vi "EQC LoadFile PixelReg.vi"(11 "PixelReg file path":path) -> (0 "Error tick":bool, 2 "PixelReg (hex)":u32[](array[numeric]) format="%x")   [LabVIEW 2015, in "VIPM2.lvlib"]
uses:
  VIPM2.lvlib
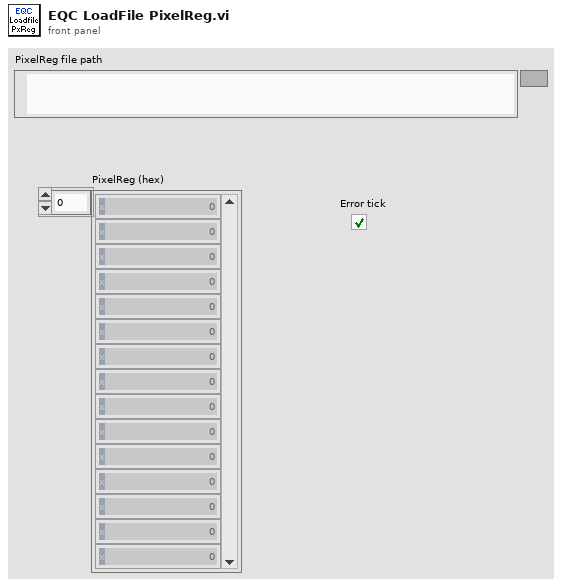
[diagram p1: front panel]
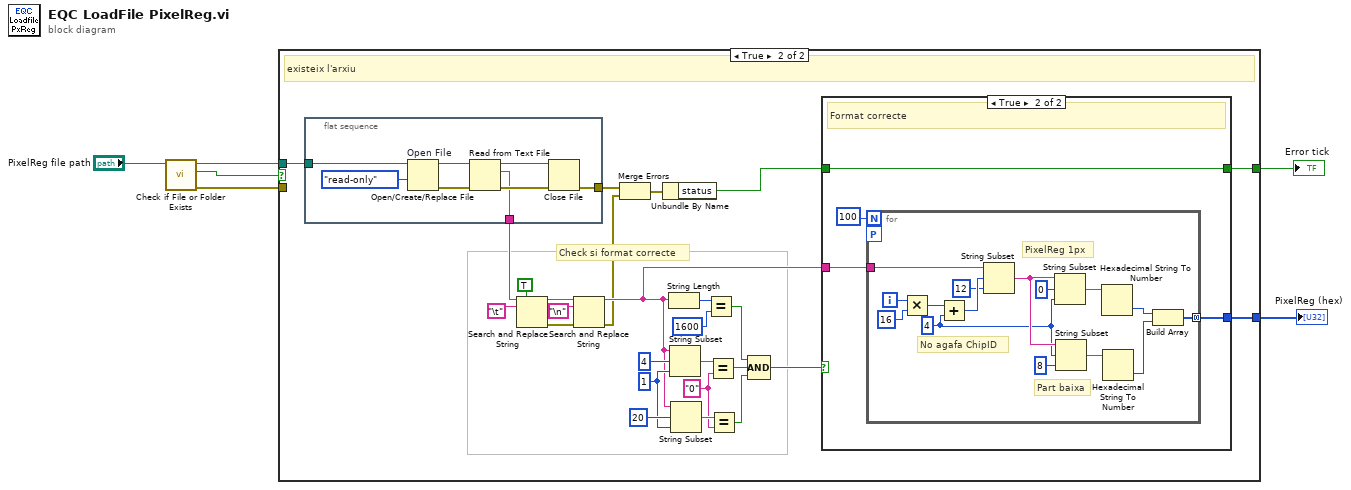
[diagram p0: block diagram]
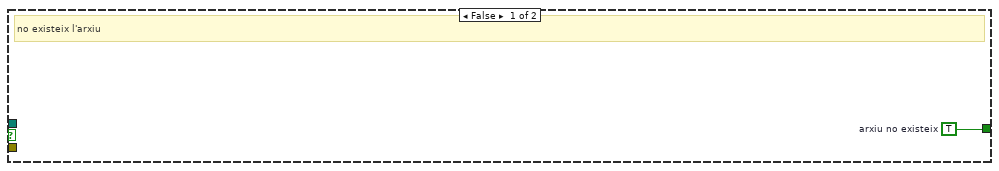
[diagram p2: hidden frame]
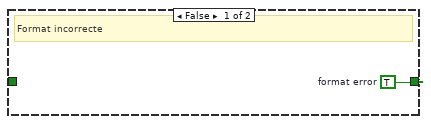
[diagram p3: hidden frame]
diagram:
  n1 = call <vilib>:"Check if File or Folder Exists.vi"("path"="PixelReg file path") -> ("error out"=w2:errorcluster, "file or folder exists?"=w1:bool, "dup path"=w4:path)  [unwired: 8 in]
  n2 = case shown="True" w1 {
    tunnel: [_ w11] -> w6
    tunnel: [w7 w10] -> w5
    tunnel: w4 -> [_ w8]
    tunnel: w2 -> [_ _]
    frame False {
      w7 = TRUE  # arxiu no existeix
      # "no existeix l'arxiu"
    }
    frame True {
      w18 = "0"
      w17 = 1 ("length (rest)")
      # "Check si format correcte"
      # "existeix l'arxiu"
      n3 = flat-sequence {
        tunnel: [w36] -> w33
        tunnel: [w35] -> w13
        tunnel: w8 -> [w34]
        frame #0 {
          n4 = Open/Create/Replace File "Open File"(file path (use dialog)=w34, access (0:read/write)=enum16{"read/write", "read-only", "write-only"}."read-only") -> (refnum out=w40:refnum<file>, error out=w41:errorcluster)  [unwired: 4 in, 1 out]
          n5 = Read from Text File(file (use dialog)=w40, error in=w41) -> (refnum out=w37:refnum<file>, text=w36:string, error out=w38:errorcluster)  [unwired: 2 in, 1 out]
          n6 = Close File(refnum=w37, error in=w38) -> (error out=w35:errorcluster)  [unwired: 1 out]
        }
      }
      n7 = Search and Replace String(replace all?=TRUE ("replace all? (F)"), input string=w33, search string="\t") -> (result string=w30:string, error out=w29:errorcluster)  [unwired: 5 in, 2 out]
      n8 = Search and Replace String(input string=w30, search string="\n", error in=w29) -> (result string=w15:string, error out=w14:errorcluster)  [unwired: 5 in, 2 out]
      n9 = Merge Errors(w13, w14) -> (w12:errorcluster)
      n10 = Unbundle By Name(w12) -> ("status"=w9:bool)
      n11 = String Length(string=w15) -> (length=w27:i32)
      n12 = String Subset(string=w15, offset (0)=4, length (rest)=w17) -> (substring=w23:string)
      n13 = String Subset(string=w15, offset (0)=20, length (rest)=w17) -> (substring=w19:string)
      n14 = Equal?(x=w27, y=1600) -> (x = y?=w21:bool)
      n15 = Equal?(x=w23, y=w18) -> (x = y?=w22:bool)
      n16 = Equal?(x=w19, y=w18) -> (x = y?=w20:bool)
      n17 = Compound Arithmetic op=AND(w21, w22, w20) -> (w16:bool)
      n18 = case shown="True" w16 {
        tunnel: w15 -> [_ w45]
        tunnel: [_ w44] -> w11
        tunnel: [w42 w43] -> w10
        tunnel: w9 -> [_ w43]
        frame False {
          w42 = TRUE  # format error
          # "Format incorrecte"
        }
        frame True {
          # "Format correcte"
          n19 = for {
            N: 100 -> [_]
            tunnel: w45 -> [w60]
            tunnel: [w47] -> w44 mode=concatenating
            workers-P: _ -> [_]
            i -> [w61]
            w53 = 4 ("y")
            # "Part baixa"
            # "PixelReg 1px"
            # "No agafa ChipID"
            n20 = Multiply(x=w61, y=16) -> (x*y=w58:i32)
            n21 = Add(x=w58, y=w53) -> (x+y=w57:i32)
            n22 = String Subset(string=w60, offset (0)=w57, length (rest)=12 ("length (rest)")) -> (substring=w54:string)
            n23 = String Subset(string=w54, offset (0)=0, length (rest)=w53) -> (substring=w51:string)
            n24 = String Subset(string=w54, offset (0)=w53, length (rest)=8 ("length (rest)")) -> (substring=w50:string)
            n25 = Hexadecimal String To Number(string=w51) -> (number=w49:u32)  [unwired: 2 in, 1 out]
            n26 = Hexadecimal String To Number(string=w50) -> (number=w48:u32)  [unwired: 2 in, 1 out]
            n27 = Build Array(w49, w48) -> (w47:u32[])
          }
        }
      }
    }
  }
  "PixelReg (hex)" <- w6
  "Error tick" <- w5
